vi "Day 4.vi"() -> ()   [LabVIEW 2020]
uses:
  <vilib>/Utility/file.llb/Read Delimited Spreadsheet (string).vi
  <userlib>/_OpenG.lib/array/array.llb/Search 1D Array (String)__ogtk.vi
panel:
  out "array":i32[](array[numeric])
  out "Bingo Cards":i32[][][](array[numeric])
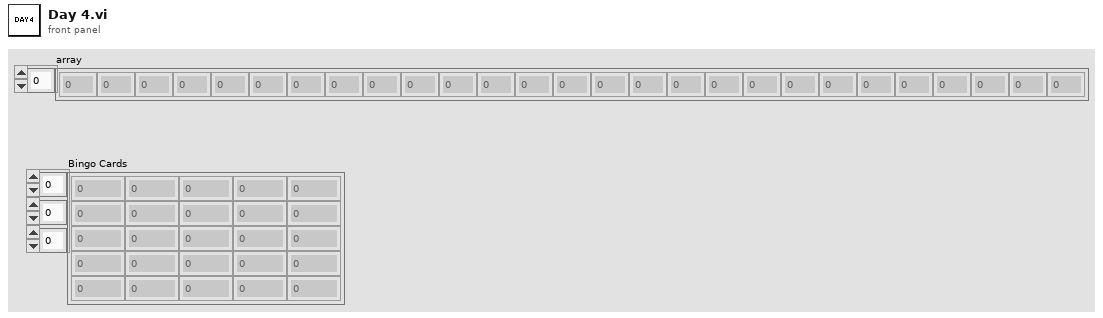
[diagram p1: front panel]
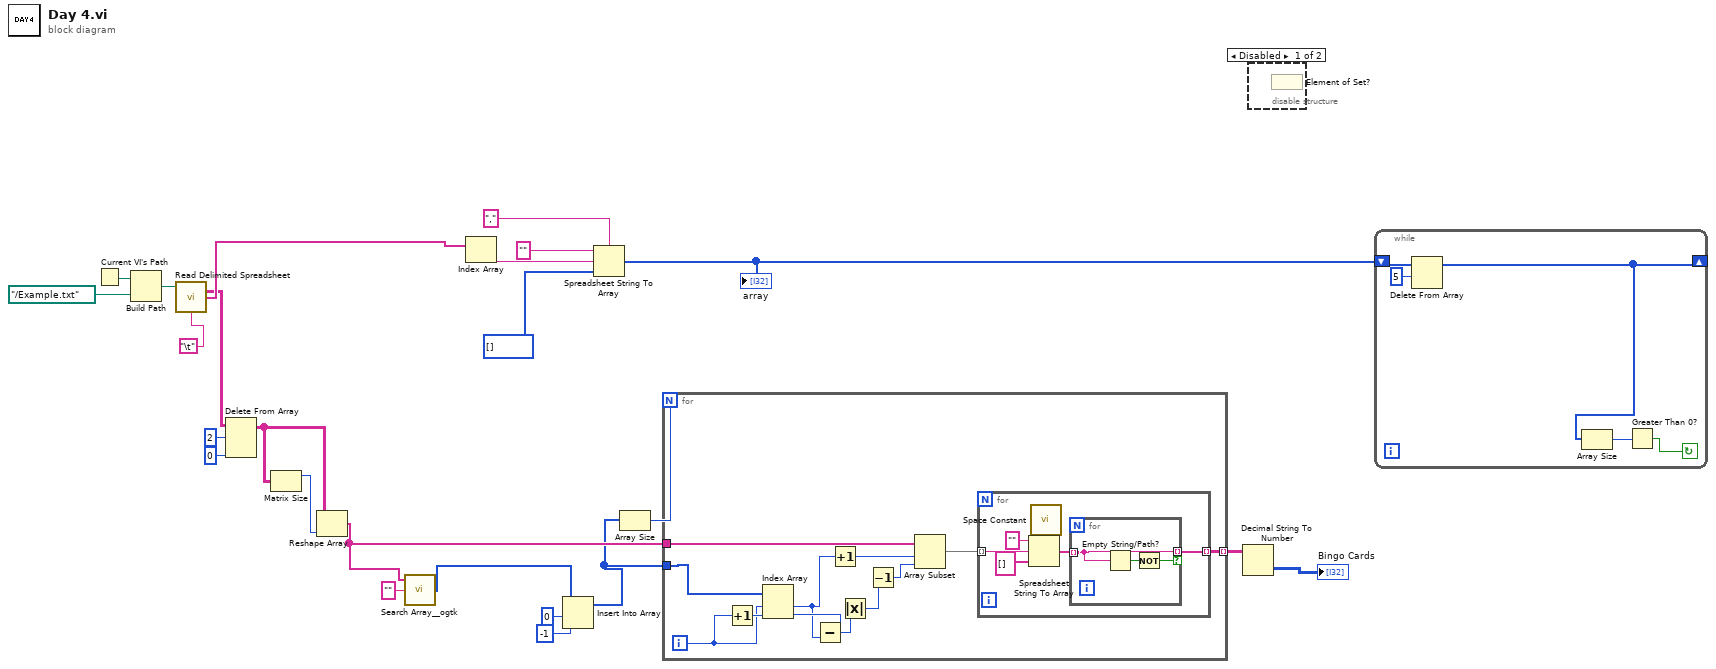
[diagram p0: block diagram]
diagram:
  n1 = Current VI's Path() -> (path=w23:path)
  n2 = Build Path(base path=w23, name or relative path=path "../Example.txt" ("file path (dialog if empty)")) -> (appended path=w21:path)
  n3 = call-poly <vilib>:"Read Delimited Spreadsheet.vi"("file path (dialog if empty)"=w21, "delimiter (\\t)"="\t") -> ("all rows"=w13:string[][], "first row"=w19:string[])  [unwired: 8 in, 4 out]
  n4 = Delete From Array(array=w13, length=2, index (row)=0 ("index")) -> (array with subset deleted=w11:string[][])  [unwired: 1 in, 1 out]
  n5 = Matrix Size(0:w11) -> (1:w12:i32)  [unwired: 1 out]
  n6 = Reshape Array(w11, w12) -> (w8:string[])
  n7 = call-poly <userlib>:"Search Array__ogtk.vi"("Array"=w8, "Element Data"="") -> ("Indices of Elements"=w5:i32[])  [unwired: 7 in]
  n8 = Index Array(array=w19) -> (element=w18:string)  [unwired: 1 in]
  n9 = Insert Into Array(array=w5, index=0, new element=-1 ("new element/subarray")) -> (w3:i32[])
  n10 = Spreadsheet String To Array(delimiter (Tab)=",", format string="", spreadsheet string=w18, array type (2D Dbl)=i32[] []) -> (array=w10:i32[])
  "array" <- w10
  n11 = Array Size(array=w3) -> (size(s)=w4:i32)
  n12 = for {
    N: w4 -> [_]
    tunnel: w8 -> [w36]
    tunnel: w3 -> [w33]
    tunnel: [w25] -> w2 mode=indexing
    i -> [w34]
    n13 = Increment(x=w34) -> (x+1=w35:i32)
    n14 = Index Array(array=w33, index #1=w34, index #2=w35) -> (element #1=w30:i32, element #2=w32:i32)
    n15 = Subtract(x=w32, y=w30) -> (x-y=w29:i32)
    n16 = Increment(x=w30) -> (x+1=w31:i32)
    n17 = Absolute Value(x=w29) -> (abs(x)=w28:i32)
    n18 = Decrement(x=w28) -> (x-1=w27:i32)
    n19 = Array Subset(array=w36, index=w31, length=w27) -> (w26:string[])
    n20 = for {
      tunnel: w26 -> [w41] mode=indexing
      tunnel: [w37] -> w25 mode=indexing
      n21 = call <vilib>:"Space Constant.vi"() -> ("String"=w42:string)
      n22 = Spreadsheet String To Array(delimiter (Tab)=w42, format string="", spreadsheet string=w41, array type (2D Dbl)=string[] []) -> (array=w38:string[])
      n23 = for {
        tunnel: w38 -> [w45] mode=indexing
        tunnel: [w45] -> w37 mode=indexing if=w43
        n24 = Empty String/Path?(string/path=w45) -> (empty?=w44:bool)
        n25 = Not(x=w44) -> (.not. x?=w43:bool)
      }
    }
  }
  n26 = Decimal String To Number(string=w2) -> (number=→"Bingo Cards":i32[][][])  [unwired: 2 in, 1 out]
  n27 = disable-structure shown="Disabled" {
    frame Disabled {
      n28 = Element of Set?() -> ()  [unwired: 2 in, 1 out]
    }
    frame Enabled {
    }
  }
  n29 = while {
    shift-right: [w47] -> _
    shift-left: w10 -> [w50]
    stop <- w48 continue-if-true
    n30 = Delete From Array(array=w50, length=5) -> (array with subset deleted=w47:i32[])  [unwired: 1 in, 1 out]
    n31 = Array Size(array=w47) -> (size(s)=w49:i32)
    n32 = Greater Than 0?(x=w49) -> (x > 0?=w48:bool)
  }
